vi "Wait Any Example.vi"() -> ()   [LabVIEW 2020, in "Futures-Examples.lvlib"]
uses:
  Futures-Examples.lvlib
  DoubleValue/DoubleValue.lvclass/DoubleValue.ctl
  Promises/Promise/Promise.lvclass/Promise.ctl
  Promises/Future/Future.lvclass/Future.ctl
  DoubleValue/DoubleValue.lvclass
  C:/dev/lv/2020/lv-promises/Promises/Value/Value.lvclass
  StringValue/StringValue.lvclass
  StringValue/StringValue.lvclass/StringValue.ctl
  Promises/Future/Future.lvclass
  Promises/Promise/Promise.lvclass
panel:
  out "Value":string
  out "Resolved Future Index":i32
  out "Resolved Error":errorcluster
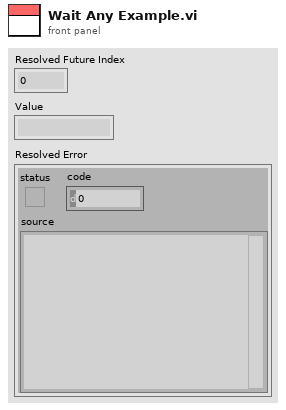
[diagram p1: front panel]
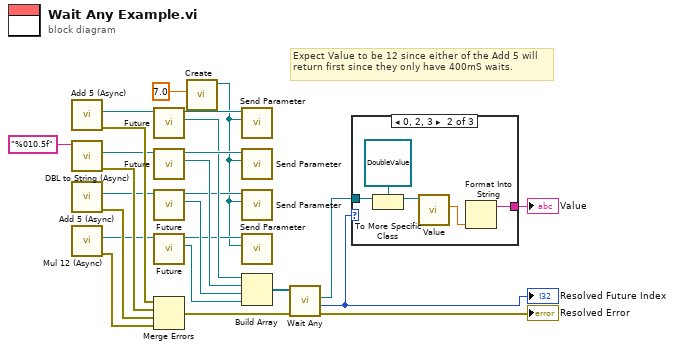
[diagram p0: block diagram]
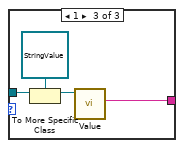
[diagram p3: hidden frame]
diagram:
  # "Expect Value to be 12 since either of the Add 5 will return first since they only have 400mS waits."
  n1 = call "Add 5 (Async).vi"() -> ("error out"=w25:errorcluster, "Add 5 Promise"=w21:refnum<class "Promise.lvclass">)  [unwired: 10 in]
  n2 = call "DBL to String (Async).vi"("Format String"="%010.5f") -> ("error out"=w24:errorcluster, "Promise out"=w16:refnum<class "Promise.lvclass">)  [unwired: 9 in]
  n3 = call "Add 5 (Async).vi"() -> ("error out"=w23:errorcluster, "Add 5 Promise"=w18:refnum<class "Promise.lvclass">)  [unwired: 10 in]
  n4 = call "Mul 12 (Async).vi"() -> ("error out"=w22:errorcluster, "Mul 12 Promise"=w17:refnum<class "Promise.lvclass">)  [unwired: 10 in]
  n5 = call "Future.vi"("Promise in"=w21) -> ("Future"=w14:refnum<class "Future.lvclass">, "Promise"=w4:refnum<class "Promise.lvclass">)  [unwired: 9 in]
  n6 = call "Future.vi"("Promise in"=w16) -> ("Future"=w11:refnum<class "Future.lvclass">, "Promise"=w15:refnum<class "Promise.lvclass">)  [unwired: 9 in]
  n7 = call "Future.vi"("Promise in"=w18) -> ("Future"=w12:refnum<class "Future.lvclass">, "Promise"=w3:refnum<class "Promise.lvclass">)  [unwired: 9 in]
  n8 = call "Future.vi"("Promise in"=w17) -> ("Future"=w13:refnum<class "Future.lvclass">, "Promise"=w2:refnum<class "Promise.lvclass">)  [unwired: 9 in]
  n9 = Merge Errors(w25, w24, w23, w22) -> (w5:errorcluster)
  n10 = call "Create.vi"("Value"=7.0) -> ("DoubleValue"=w1:refnum<class "DoubleValue.lvclass">)  [unwired: 10 in]
  n11 = call "Send Parameter.vi"("Parameter"=w1, "Promise in"=w4) -> ()  [unwired: 8 in, 2 out]
  n12 = call "Send Parameter.vi"("Parameter"=w1, "Promise in"=w15) -> ()  [unwired: 8 in, 2 out]
  n13 = call "Send Parameter.vi"("Parameter"=w1, "Promise in"=w3) -> ()  [unwired: 8 in, 2 out]
  n14 = call "Send Parameter.vi"("Parameter"=w1, "Promise in"=w2) -> ()  [unwired: 8 in, 2 out]
  n15 = Build Array(w14, w11, w12, w13) -> (w10:refnum<class "Future.lvclass">[])
  n16 = call "Wait Any.vi"("error in (no error)"=w5, "Futures"=w10) -> ("error out"=→"Resolved Error":errorcluster, "Index"=w7:i32, "Result"=w8:refnum<class "Value.lvclass">)  [unwired: 7 in]
  "Resolved Future Index" <- w7
  n17 = case shown="0, 2, 3" w7 {
    tunnel: w8 -> [_ w30 w34]
    tunnel: [_ w26 w31] -> w6
    frame Default {
    }
    frame 0, 2, 3 {
      n18 = To More Specific Class(target class=refnum<class "DoubleValue.lvclass"> refnum ("Futures-Examples.lvlib:DoubleValue.lvclass"), reference=w30) -> (specific class reference=w28:refnum<class "DoubleValue.lvclass">)  [unwired: 1 in, 1 out]
      n19 = call "Value.vi"("DoubleValue in"=w28) -> ("Value"=w27:dbl)  [unwired: 10 in]
      n20 = Format Into String(w27) -> (resulting string=w26:string)  [unwired: 3 in, 1 out]
    }
    frame 1 {
      n21 = To More Specific Class(target class=refnum<class "StringValue.lvclass"> refnum ("Futures-Examples.lvlib:StringValue.lvclass"), reference=w34) -> (specific class reference=w32:refnum<class "StringValue.lvclass">)  [unwired: 1 in, 1 out]
      n22 = call "Value.vi"("StringValue in"=w32) -> ("Value"=w31:string)  [unwired: 10 in]
    }
  }
  "Value" <- w6
